vi "run.create.path.vi"(8 "error in":errorcluster) -> (0 "error out":errorcluster, 3 "path":string)   [LabVIEW 2020, in "Nominal Client.lvclass"]
uses:
  Nominal Client.lvclass
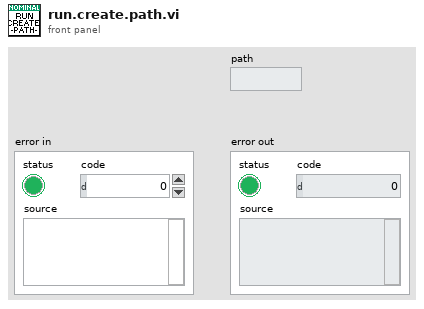
[diagram p1: front panel]
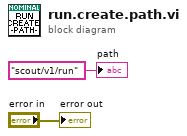
[diagram p0: block diagram]
diagram:
  "path" <- "scout/v1/run" ("Path")
  "error out" <- "error in"
